vi "effectiveglobals.vi"() -> ()   [LabVIEW 2013]
panel:
  out "Flowrate B":dbl format="%_6f"
  out "Flowrate A":dbl format="%_6f"
  out "Pressure B":dbl format="%_6f"
  out "Pressure A":dbl format="%_6f"
  out "DeltaP":dbl format="%_6f"
  out "Thickness":dbl format="%_6f"
  out "offset x1":dbl format="%_6f"
  out "Zero x":dbl format="%_6f"
  out "Porosity":dbl format="%_6f"
  out "AUX12(ch15)":dbl format="%_6f"
  out "AUX11CH14)":dbl format="%_6f"
  out "Aux10(ch13)":dbl format="%_6f"
  out "AUX9(ch12)":dbl format="%_6f"
  out "AUX8(ch11)":dbl format="%_6f"
  out "AUX7(ch10)":dbl format="%_6f"
  out "PoreADCDT":dbl format="%_6f"
  out "VerDCDT":dbl format="%_6f"
  out "ConfDCDT":dbl format="%_6g"
  out "Ver LOAD":dbl format="%_6f"
  out "NorDcDT":dbl format="%_6f"
  out "PoreBDCDT":dbl format="%_6f"
  out "Pore B":dbl format="%_6f"
  out "Pore A":dbl format="%_6f"
  out "Confine":dbl format="%_6f"
  out "NorLoad":dbl format="%_6f"
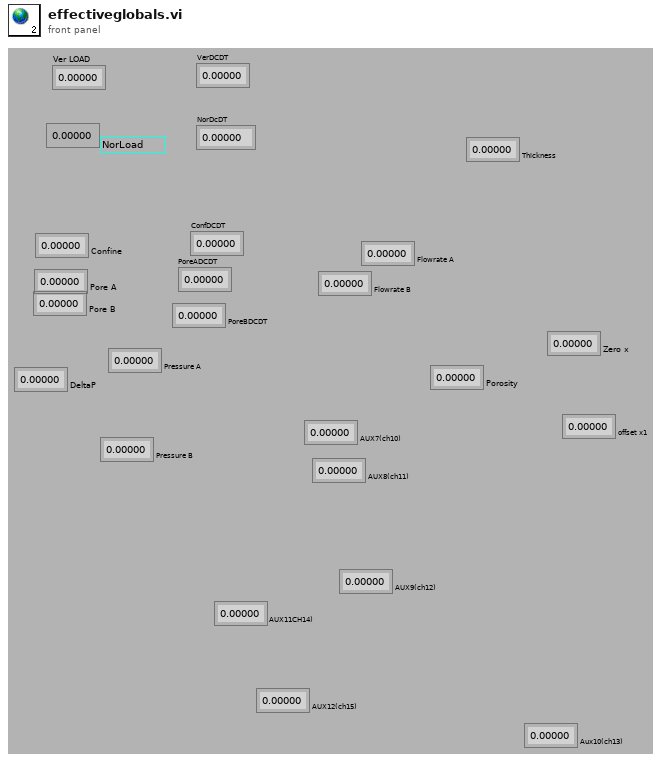
[diagram p1: front panel]
diagram:
